vi "MulDvi.vi"() -> ()   [LabVIEW 2014]
doc: "Use this template to build a VI to use as a subVI."
uses:
  <vilib>/vision/NI_Vision_Development_Module.lvlib
panel:
  out "Src":T1(plugin-control)
  out "Dst":T1(plugin-control)
  # ":: MVi Framework V1.0 ::\nAuthor:Gaoke Yang\nEmail: gaoke.yang@yahoo.com\nWeb: www.mvicontrol.com\nCopyright (C) 2015, MVI Technologies All Rights Reserved"
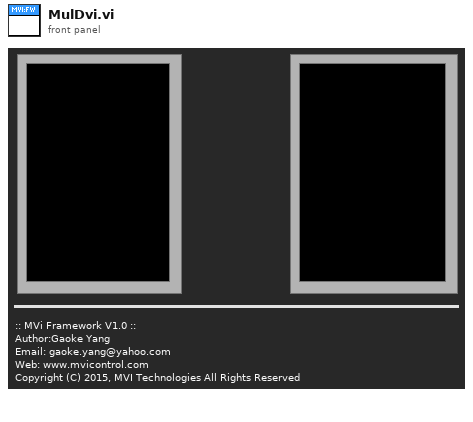
[diagram p1: front panel]
types:
  T1 = typedef "IMAQ Image.ctl" = refnum<image>
  T2 = typedef "Image Type" = u32
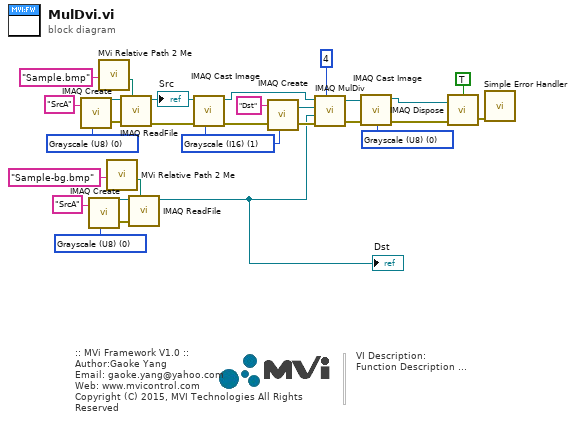
[diagram p0: block diagram]
diagram:
  w7 = T2 0 items=["Grayscale (U8)", "Grayscale (I16)", "Grayscale (SGL)", "Complex (CSG)", "RGB (U32)", "HSL (U32)", "RGB (U64)", "Grayscale (U16)"] ("Image Type")
  w11 = T2 0 items=["Grayscale (U8)", "Grayscale (I16)", "Grayscale (SGL)", "Complex (CSG)", "RGB (U32)", "HSL (U32)", "RGB (U64)", "Grayscale (U16)"] ("Image Type")
  w10 = T2 1 items=["Grayscale (U8)", "Grayscale (I16)", "Grayscale (SGL)", "Complex (CSG)", "RGB (U32)", "HSL (U32)", "RGB (U64)", "Grayscale (U16)"] ("Image Type")
  w22 = T2 0 items=["Grayscale (U8)", "Grayscale (I16)", "Grayscale (SGL)", "Complex (CSG)", "RGB (U32)", "HSL (U32)", "RGB (U64)", "Grayscale (U16)"] ("Image Type")
  # "VI Description:\nFunction Description ..."
  # ":: MVi Framework V1.0 ::\nAuthor:Gaoke Yang\nEmail: gaoke.yang@yahoo.com\nWeb: www.mvicontrol.com\nCopyright (C) 2015, MVI Technologies All Rights Reserved"
  n1 = call "IMAQ Create"("Image Name"="SrcA" ("name or relative path"), "Image Type"=w22) -> ("New Image"=w23:T1, "error out"=w21:errorcluster)  [unwired: 2 in, 1 out]
  n2 = call "IMAQ Create"("Image Name"="SrcA" ("name or relative path"), "Image Type"=w7) -> ("New Image"=w6:T1, "error out"=w8:errorcluster)  [unwired: 2 in, 1 out]
  n3 = call "MVi Relative Path 2 Me.vi"("Relative Path"="Sample.bmp" ("name or relative path")) -> ("Appended Dir"=w25:path)  [unwired: 5 in, 1 out]
  n4 = call "MVi Relative Path 2 Me.vi"("Relative Path"="Sample-bg.bmp" ("name or relative path")) -> ("Appended Dir"=w5:path)  [unwired: 5 in, 1 out]
  n5 = call "IMAQ ReadFile"("File Path"=w25, "error in (no error)"=w21, "Image"=w23) -> ("error out"=w17:errorcluster, "Image Out"=w9:T1)  [unwired: 4 in, 3 out]
  "Src" <- w9
  n6 = call "IMAQ ReadFile"("File Path"=w5, "error in (no error)"=w8, "Image"=w6) -> ("Image Out"=w1:T1)  [unwired: 4 in, 4 out]
  "Dst" <- w1
  n7 = call "IMAQ Cast Image"("Image Type"=w10, "error in (no error)"=w17, "Image Src"=w9) -> ("error out"=w16:errorcluster, "Image Dst Out"=w15:T1)  [unwired: 7 in]
  n8 = call "IMAQ Create"("Image Name"="Dst" ("name or relative path"), "Image Type"=w10, "error in (no error)"=w16) -> ("New Image"=w19:T1, "error out"=w20:errorcluster)  [unwired: 1 in, 1 out]
  n9 = call "IMAQ MulDiv"("Image Src A"=w15, "Constant"=i8 4, "Image Dst"=w19, "Image Src B"=w1, "error in (no error)"=w20) -> ("Image Dst Out"=w13:T1, "error out"=w14:errorcluster)  [unwired: 2 in]
  n10 = call "IMAQ Cast Image"("Image Type"=w11, "error in (no error)"=w14, "Image Src"=w13) -> ("error out"=w12:errorcluster, "Image Dst Out"=w2:T1)  [unwired: 7 in]
  n11 = call "IMAQ Dispose"("All Images? (No)"=TRUE, "Image"=w2, "error in (no error)"=w12) -> ("error out"=w26:errorcluster)  [unwired: 3 out]
  n12 = call <vilib>:"Simple Error Handler.vi"("error in (no error)"=w26) -> ()  [unwired: 1 in, 8 out]
